vi "FIFOs.vi"() -> ()   [LabVIEW 2015]
panel:
  out "Array":refnum<k21>[][][](array[refnum])
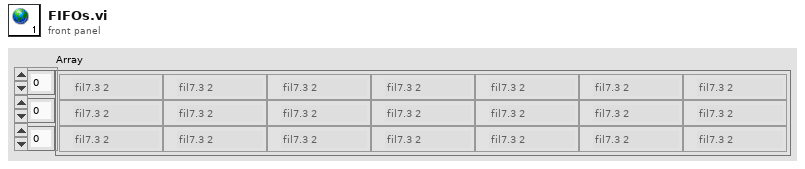
[diagram p1: front panel]
diagram:
